vi "Waveform and Laser Controls V6.vi"() -> ()   [LabVIEW 2014]
uses:
  Waveform Scan Parameters.ctl
  <vilib>/Platform/TimedLoop/XDataNode/timing_clust.ctl
  <vilib>/Platform/TimedLoop/XDataNode/nitl_modes.ctl
  <vilib>/Platform/TimedLoop/XDataNode/wakeup.ctl
  <vilib>/rvi/Emulation/niFpgaGetClockAttributes.vi
  <vilib>/rvi/Emulation/niFpgaSctlEmulationGetInTimedLoop.vi
  <vilib>/rvi/Emulation/niFpgaEmulationReportErrorSimple.vi
  <vilib>/rvi/Emulation/niFpgaProcessEmulError.vi
  <vilib>/rvi/eio/common/nirviEmuTemplateMethod_errors.vi
  <vilib>/rvi/Emulation/niFpgaCriticalErrorInLSC.vi
  <vilib>/rvi/Memory/Memory_Emulation/nirvimemoryFastEmulation.vi
  <vilib>/rvi/Memory/Memory_Emulation/nirvimemoryEmulation.vi
  <vilib>/rvi/Emulation/niFpgaEmulationIsFPGAContextNoSignature.vi
  <vilib>/rvi/DataTransferAndStorage/Container/Common/niFpgaContainerGetUniqueNameForEmu.vi
  <vilib>/rvi/errors/nirviReportUnexpectedCaseInternalError (U32).vi
  <vilib>/rvi/Memory/Memory_Emulation/niFpgaMemoryEmulationCacheClearOnFirstRun.vi
  <vilib>/rvi/Memory/Memory_Emulation/nirvimemoryEmulationManagerCache_MakeExclusive.vi
  <vilib>/rvi/Memory/Memory_Emulation/niFpgaMemoryEmulationValidateCache.vi
  <vilib>/rvi/Memory/Memory_Emulation/nirvimemoryEmulationManagerCache_InsertValue.vi
  <vilib>/Utility/error.llb/Clear Errors.vi
  <vilib>/rvi/Memory/Memory_Emulation/nirvimemoryEmulationManagerCache_ReleaseExclusive.vi
  <vilib>/rvi/Memory/Memory_Emulation/nirvimemoryEmulationManagerCache_GetValue.vi
  <vilib>/rvi/Memory/Memory_Emulation/nirvimemoryEmulationManagerCache_SetValue.vi
  <vilib>/eio/EIONode/EIONode.xnode
  <vilib>/rvi/DataTransferAndStorage/Container/XNode/niFpgaContainer.xnode
  <vilib>/Platform/TimedLoop/XDataNode/XDataNode.xnode
  <vilib>/rvi/DataTransferAndStorage/Register/Emulation/niFpgaRegisterEmulation.vi
  <vilib>/Platform/TimedLoop/XDataNode/XDNodeRunTimeDep.lvlib
panel:
  in  "Current Frame":u8
  in  "Lower Shutter Command":bool
  in  "Upper Shutter Command":bool
  out "Lower Shutter Status":bool
  out "Upper Shutter Status":bool
  in  "stop":bool
  in  "775 AOM (I16)":i16=16500
  out "Laser Blank Trigger":bool
  in  "Laser On Time (Ticks)":u8=8
  in  "Sequences":u8=4
  in  "Laser Delay (Ticks)":u8
  in  "Laser States":u32
  in  "Blanking Off/Manual":bool
  in  "Z Piezo Axis":i16
  in  "Y Piezo Axis":i16
  in  "X Piezo Axis":i16
  out "End Linear Ramp":bool
  in  "End of Linear Ramp":u32
  in  "Z Stack Start Position (I16)":i16
  in  "Frames Per Z Step":u8
  in  "Number of Z Steps":u8
  in  "Z Step Size (I16)":i16
  in  "Stop Sync Signal":bool
  in  "Accums Per Line":u32[](array[numeric])=[0, 0, 0, 0]
  in  "Number of Lines":u32
  out "Frame Trigger":bool
  in  "Reset Position Error":bool
  in  "Galvo 1 Position (I16)":i16
  in  "Galvo 2 Position (I16)":i16
  in  "WF 3 Data Loaded":bool
  in  "WF 2 Data Loaded":bool
  in  "Waveform Scan Parameters":T1={"Scanning Mode"=0, "Fast Axis WF Length (Elements)"=0, "Fast Axis Sample Period (Ticks)"=40, "Slow Axis 1 WF Length (Elements)"=0, "Slow Axis 1 Sample Period (Ticks)"=40, "Slow Axis 1 Delay (25 ns) Steps"=40, "Slow Axis 2 WFLength (Elements)"=0, "Slow Axis 2 Sample Period (Ticks)"=40, "Slow Axis 2 Delay (25 ns) Steps"=40}
  in  "Resonant Mirror":T2
  in  "Galvo Mirror 2":T3
  in  "Galvo Mirror 1":T3
  in  "Start Waveforms":bool
  in  "Unused Axis Offset":i16
  in  "Slow Axis 2 Waveform Element":i16
  in  "Fast Axis Waveform Element":i16
  in  "Slow Axis 1 Waveform Element":i16
  in  "WF 1 Data Loaded":bool
  # "V2 - Adding in a line clock\nV3 - Cluster Scan Parameters"
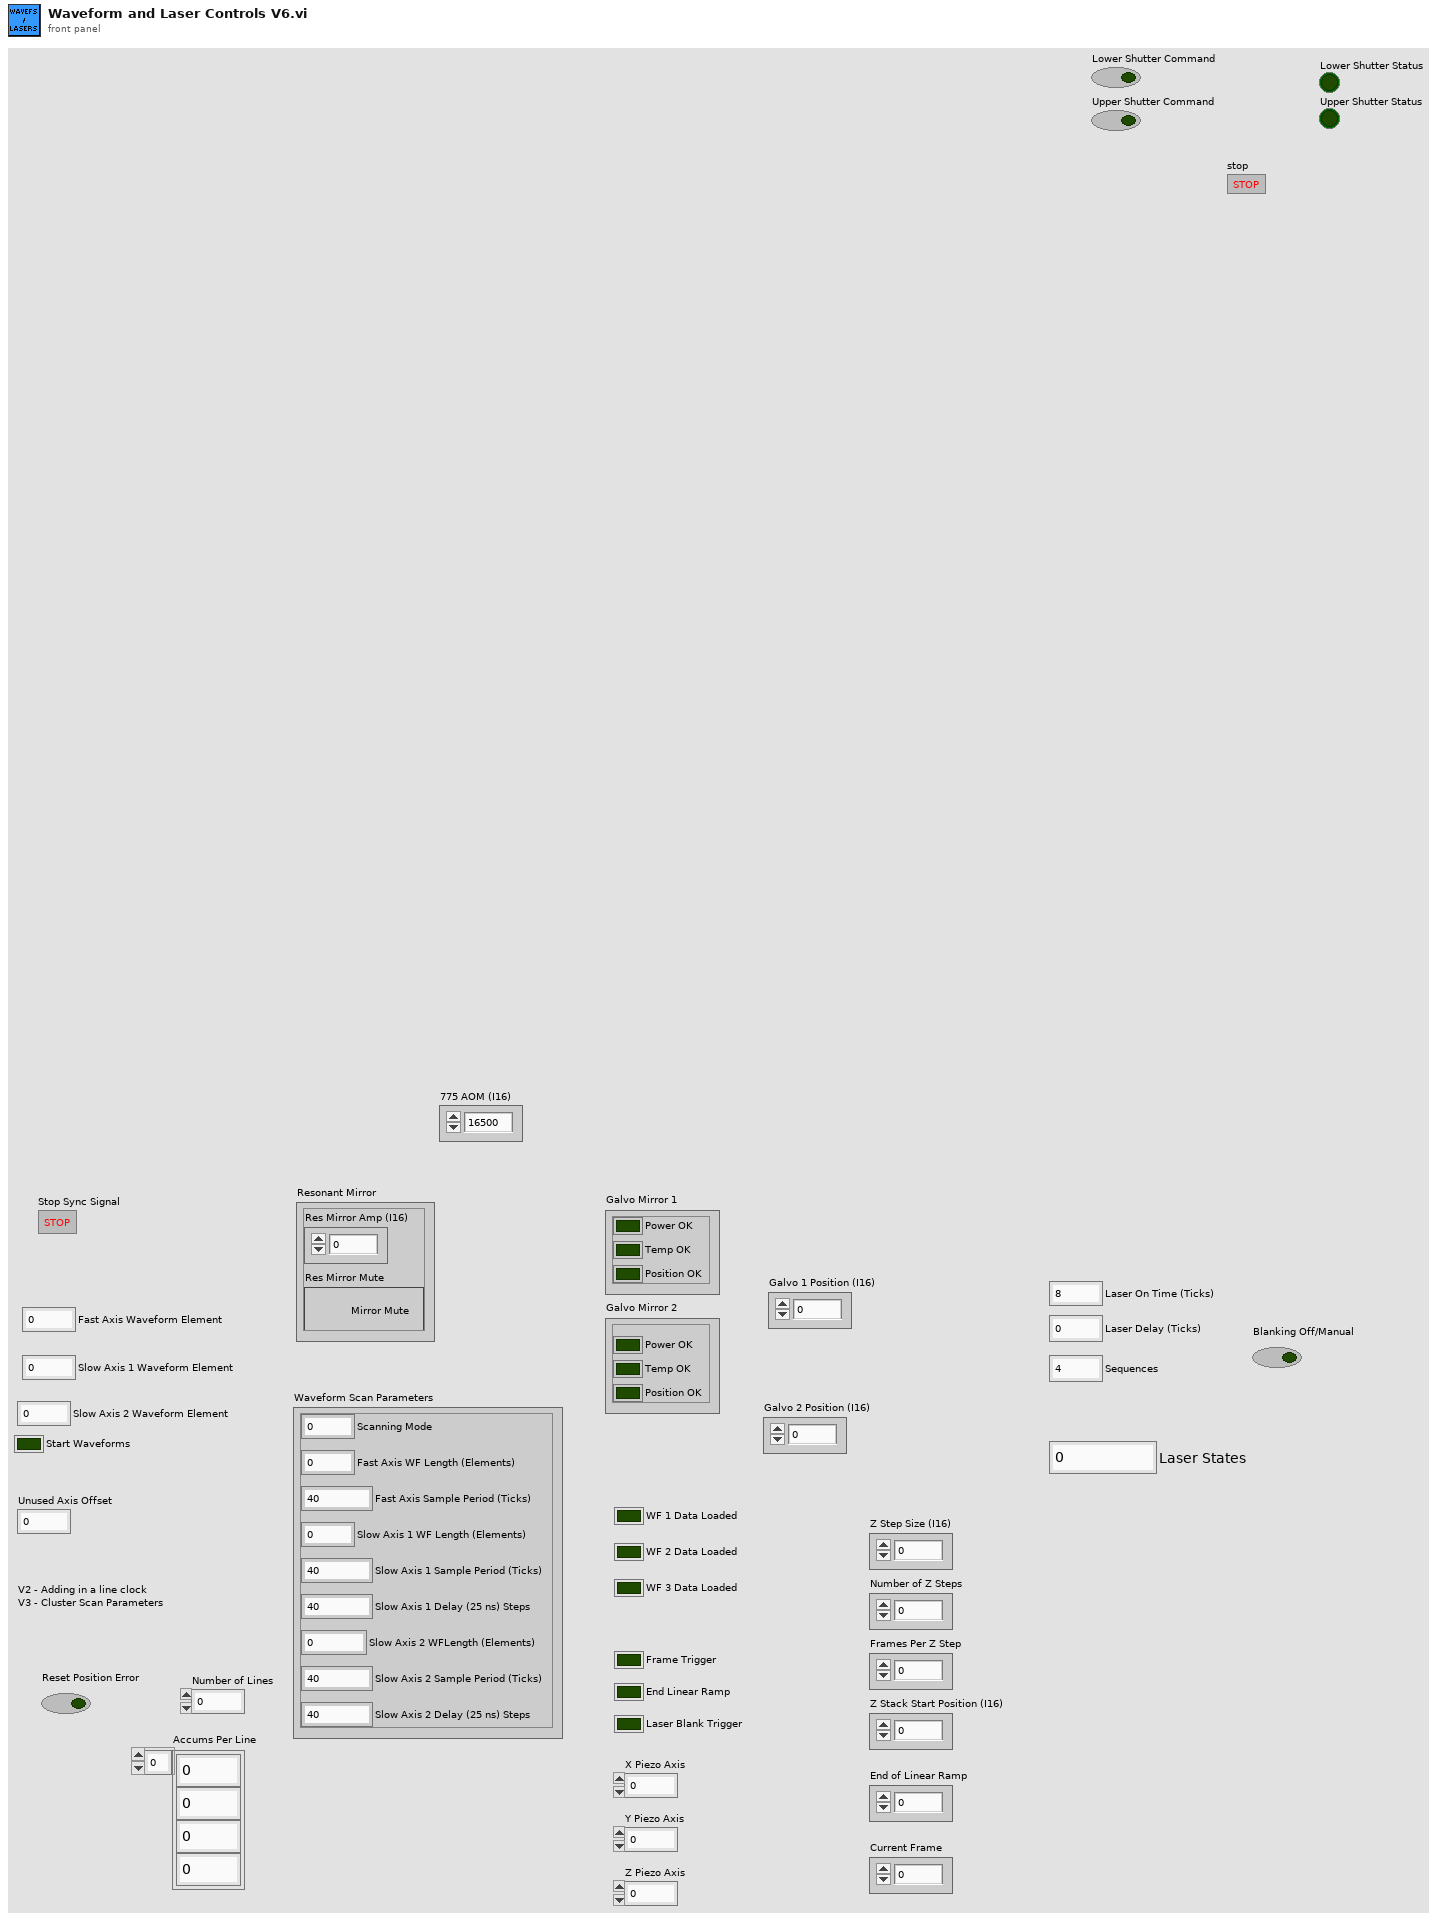
[diagram p1: front panel]
types:
  T1 = typedef "Waveform Scan Parameters.ctl" = cluster{"Scanning Mode":u8, "Fast Axis WF Length (Elements)":i32, "Fast Axis Sample Period (Ticks)":u32, "Slow Axis 1 WF Length (Elements)":i32, "Slow Axis 1 Sample Period (Ticks)":u32, "Slow Axis 1 Delay (25 ns) Steps":i32, "Slow Axis 2 WFLength (Elements)":i32, "Slow Axis 2 Sample Period (Ticks)":u32, "Slow Axis 2 Delay (25 ns) Steps":i32}
  T2 = cluster{"Res Mirror Amp (I16)":i16, "Res Mirror Mute":bool}
  T3 = cluster{"Power OK":bool, "Temp OK":bool, "Position OK":bool}
  T4 = typedef "XDNodeRunTimeDep.lvlib/timing_clust.ctl" = cluster{"Expected End [f-1]":u64, "Actual End [f-1]":u64, "Finished Late? [f-1]":bool, "Expected End [i-1]":u64, "Actual End [i-1]":u64, "Finished Late? [i-1]":bool, "Expected Start [i]":u64, "Actual Start [i]":u64, "Expected Start [f]":u64, "Actual Start [f]":u64, "Source Name":string, "Structure Name":string, "Period":i64, "Deadline":i64, "Offset":i64, "Start":i64, "Priority":i32, "Timeout":i32, "Mode":T5, "Wakeup Reason":T6, "Error":errorcluster, "Source Type":string, "Secondary Source Type":string, "Global End Time":u64, "Global Start Time":u64, "Frame Duration":u64, "Iteration Duration":u64, "Assigned CPU":i32, "I/O Scan Engine Mode":u32}
  T5 = typedef "XDNodeRunTimeDep.lvlib/nitl_modes.ctl" = enum32{"No Change", "Process missed periods, maintain original phase", "Discard missed periods, maintain original phase", "Process missed periods, ignore original phase", "Discard missed periods, ignore original phase"}
  T6 = typedef "XDNodeRunTimeDep.lvlib/wakeup.ctl" = enum32{"Normal", "Aborted", "Asynchronous wakeup", "Timing source error", "Timed loop error", "Timeout"}
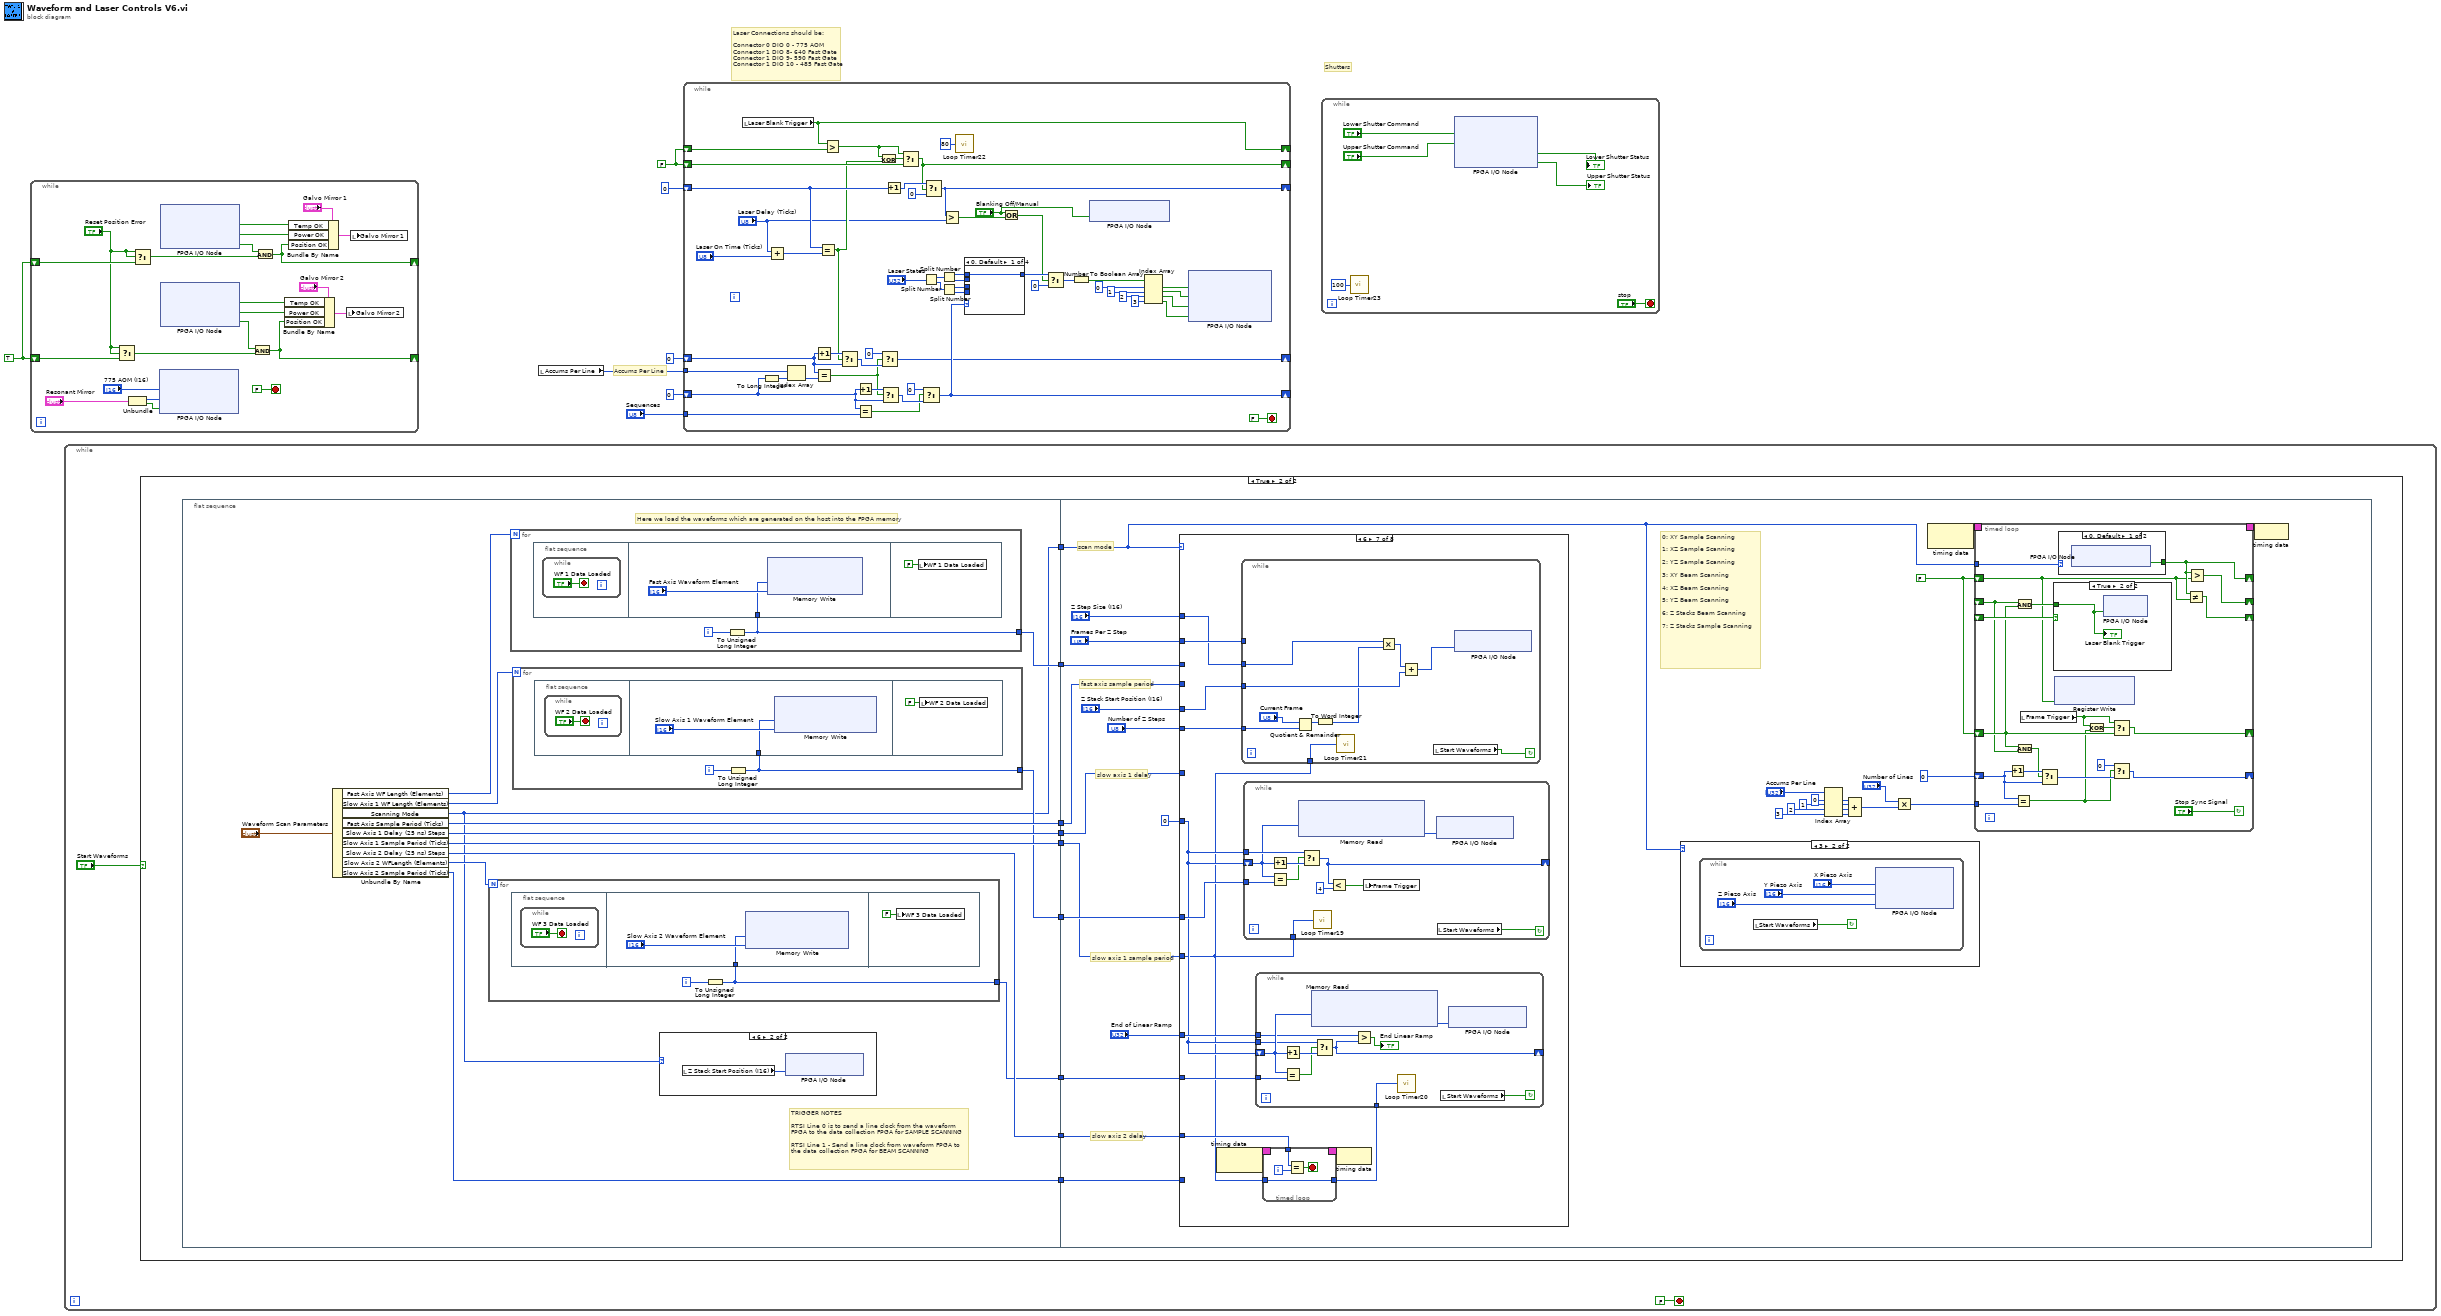
[diagram p0: block diagram]
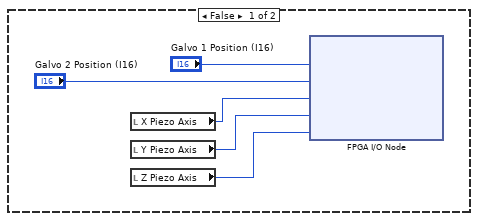
[diagram p5: hidden frame]
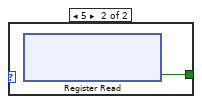
[diagram p7: hidden frame]
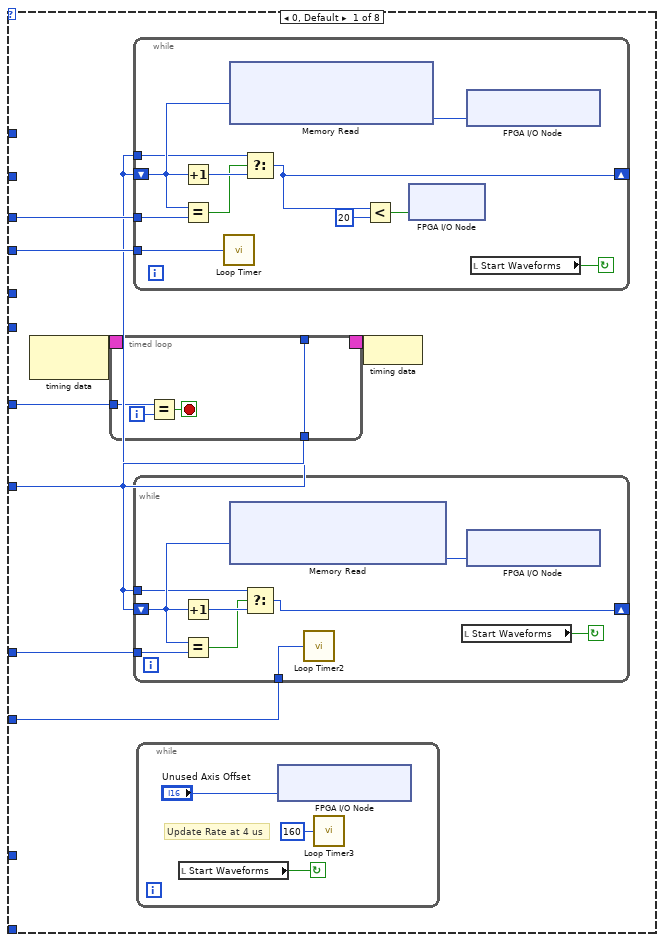
[diagram p10: hidden frame]
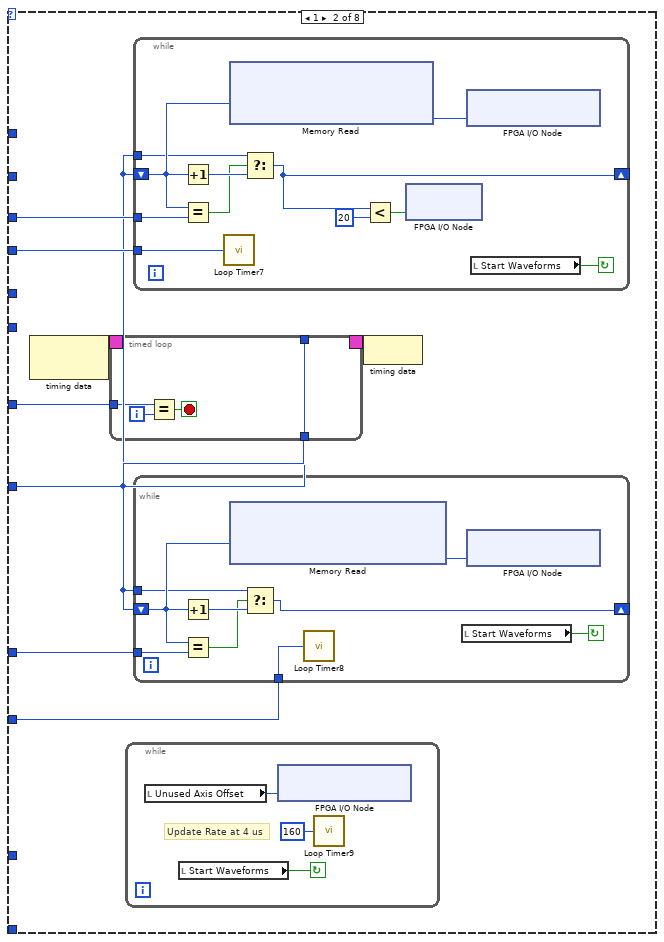
[diagram p11: hidden frame]
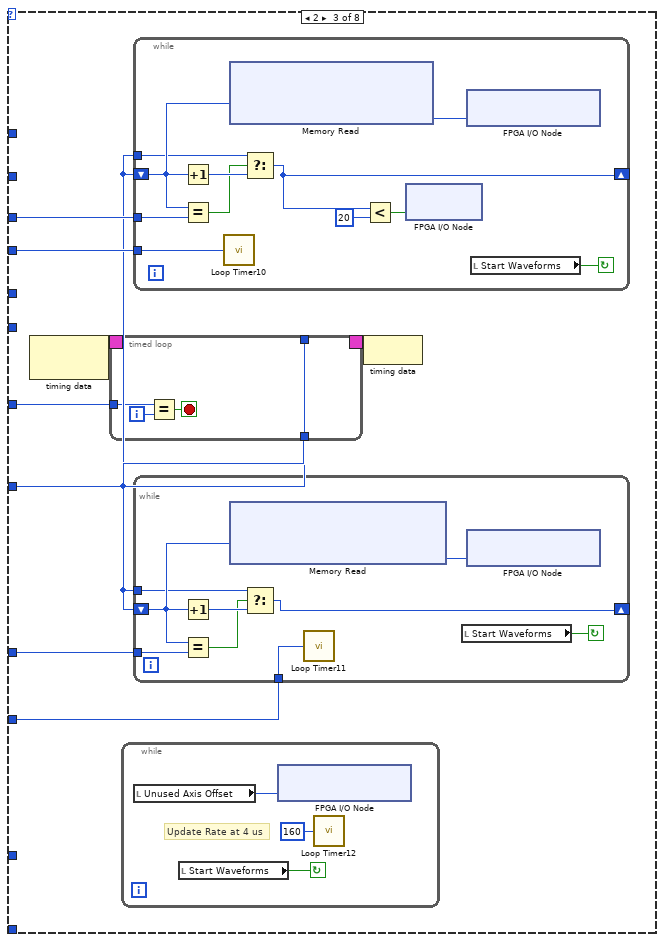
[diagram p12: hidden frame]
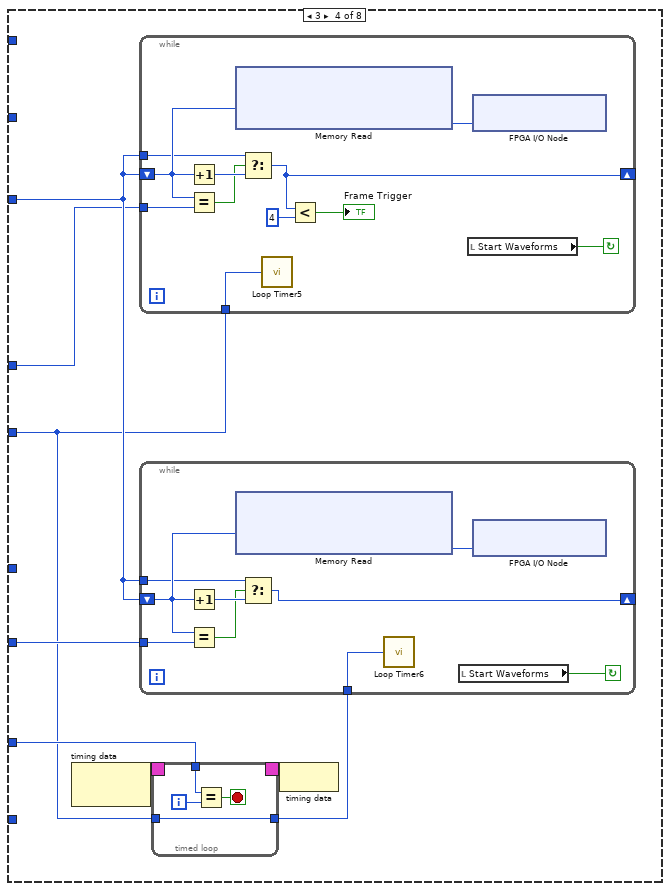
[diagram p13: hidden frame]
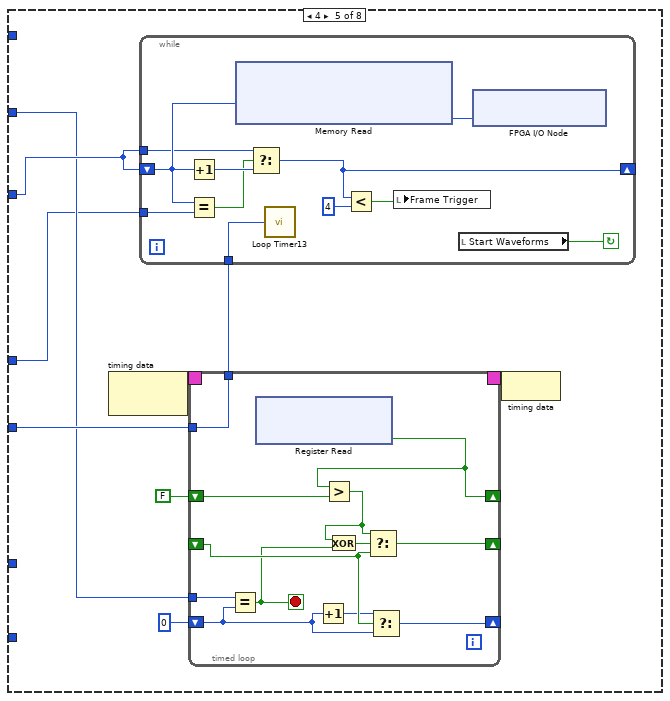
[diagram p14: hidden frame]
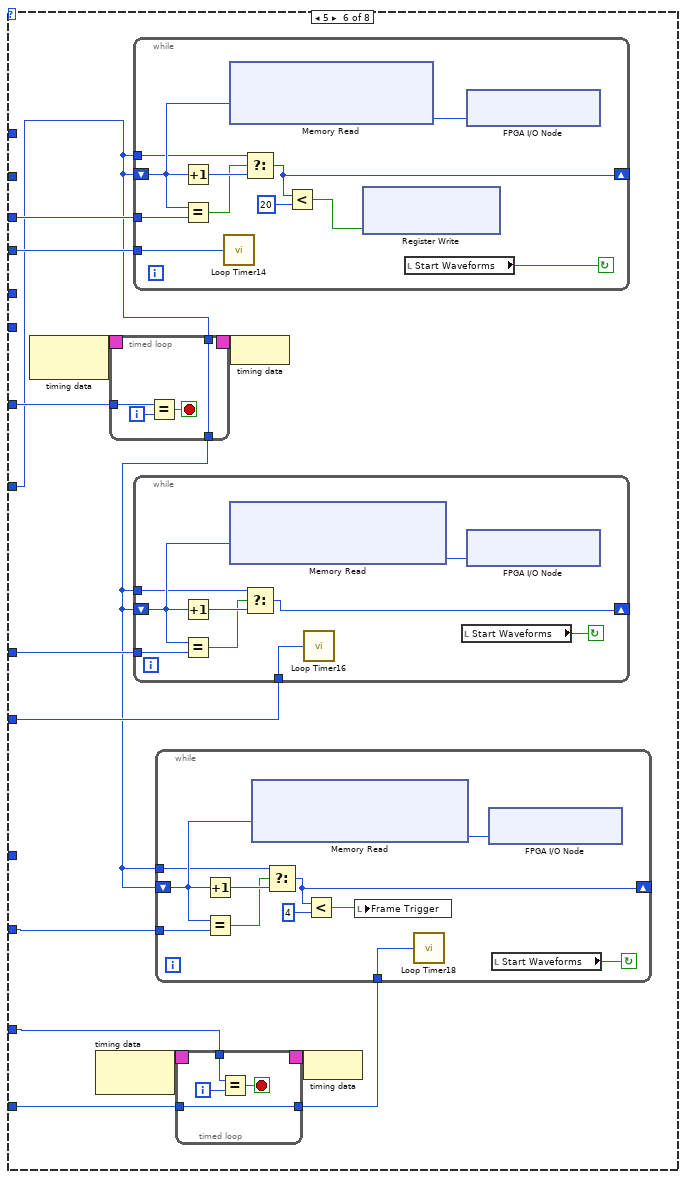
[diagram p15: hidden frame]
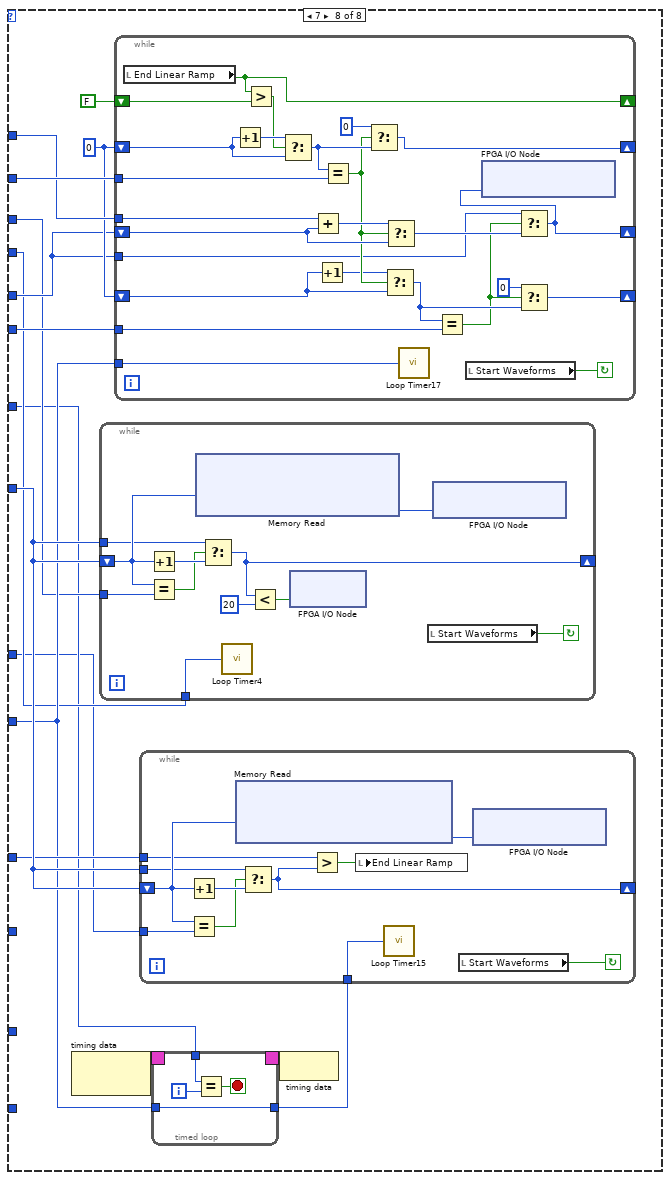
[diagram p16: hidden frame]
diagram:
  w2 = FALSE
  w7 = TRUE
  # "Shutters"
  # "Laser Connections should be:\n\nConnector 0 DIO 0 - 775 AOM\nConnector 1 DIO 8- 640 Fast Gate\nConnector 1 DIO 9- 590 Fast Gate\nConnector 1 DIO 10 - 485 Fast Gate"
  # "Accums Per Line"
  n1 = while {
    shift-right: [w15] -> _
    shift-left: w7 -> [w17]
    shift-right: [w11] -> _
    shift-left: w7 -> [w13]
    stop <- FALSE stop-if-true
    n2 = Select(t="Reset Position Error", s="Reset Position Error", f=w17) -> (s? t:f=w16:bool)
    n3 = Unbundle("Resonant Mirror") -> ("Res Mirror Amp (I16)"=w27:i16, "Res Mirror Mute"=w26:bool)
    n4 = Select(t="Reset Position Error", s="Reset Position Error", f=w13) -> (s? t:f=w12:bool)
    n5 = xnode "FPGA I/O Node"("Connector0/AO4"="775 AOM (I16)", "Connector0/AO7"=w27, "Connector0/DIO7"=w26) -> ()  [unwired: 4 in, 4 out]
    n6 = xnode "FPGA I/O Node"() -> ("Connector0/DIO1"=w8:bool, "Connector0/DIO2"=w25:bool, "Connector0/DIO3"=w14:bool)  [unwired: 4 in, 4 out]
    n7 = xnode "FPGA I/O Node"() -> ("Connector0/DIO4"=w19:bool, "Connector0/DIO5"=w20:bool, "Connector0/DIO6"=w18:bool)  [unwired: 4 in, 4 out]
    n8 = And(x=w18, y=w16) -> (x .and. y?=w15:bool)
    n9 = And(x=w14, y=w12) -> (x .and. y?=w11:bool)
    n10 = Bundle By Name(cluster="Galvo Mirror 2", "Temp OK"=w19, "Power OK"=w20, "Position OK"=w15) -> (w22:T3)
    n11 = Bundle By Name(cluster="Galvo Mirror 1", "Temp OK"=w8, "Power OK"=w25, "Position OK"=w11) -> (w24:T3)
    n12 = local write "Galvo Mirror 2"(w22) -> ()
    n13 = local write "Galvo Mirror 1"(w24) -> ()
  }
  n14 = while {
    stop <- FALSE stop-if-true
    n15 = case shown="True" "Start Waveforms" {
      frame False {
        n16 = local read "X Piezo Axis"() -> (w34:i16)
        n17 = local read "Y Piezo Axis"() -> (w33:i16)
        n18 = local read "Z Piezo Axis"() -> (w32:i16)
        n19 = xnode "FPGA I/O Node"("Connector0/AO5"="Galvo 1 Position (I16)", "Connector0/AO6"="Galvo 2 Position (I16)", "Connector0/AO1"=w34, "Connector0/AO2"=w33, "Connector0/AO3"=w32) -> ()  [unwired: 5 in, 5 out]
      }
      frame True {
        n20 = flat-sequence {
          tunnel: [w58] -> w45
          tunnel: [w48] -> w44
          tunnel: [w49] -> w43
          tunnel: [w47] -> w42
          tunnel: [w56] -> w41
          tunnel: [w55] -> w40
          tunnel: [w54] -> w39
          tunnel: [w53] -> w38
          tunnel: [w46] -> w37
          tunnel: w45 -> [w108]
          tunnel: w44 -> [w107]
          tunnel: w43 -> [w105]
          tunnel: w42 -> [w79]
          tunnel: w41 -> [w104]
          tunnel: w40 -> [w103]
          tunnel: w39 -> [w102]
          tunnel: w38 -> [w101]
          tunnel: w37 -> [w78]
          frame #0 {
            # "TRIGGER NOTES\n\nRTSI Line 0 is to send a line clock from the waveform\nFPGA to the data collection FPGA for SAMPLE SCANNING\n\nRTSI Line 1 - Send a line clock from waveform FPGA to\nthe data collection FPGA for BEAM SCANNING"
            # "Here we load the waveforms which are generated on the host into the FPGA memory"
            n21 = Unbundle By Name("Waveform Scan Parameters") -> ("Fast Axis WF Length (Elements)"=w52:i32, "Slow Axis 1 WF Length (Elements)"=w51:i32, "Scanning Mode"=w47:u8, "Fast Axis Sample Period (Ticks)"=w56:u32, "Slow Axis 1 Delay (25 ns) Steps"=w55:i32, "Slow Axis 1 Sample Period (Ticks)"=w54:u32, "Slow Axis 2 Delay (25 ns) Steps"=w53:i32, "Slow Axis 2 WFLength (Elements)"=w50:i32, "Slow Axis 2 Sample Period (Ticks)"=w46:u32)
            n22 = for {
              N: w50 -> [_]
              tunnel: [w60] -> w48
              i -> [w61]
              n23 = flat-sequence {
                tunnel: w60 -> [w63]
                frame #0 {
                  n24 = while {
                    stop <- "WF 3 Data Loaded" stop-if-true
                  }
                }
                frame #1 {
                  n25 = xnode ("Memory Write")("Address"=w63, "Data"="Slow Axis 2 Waveform Element") -> ()  [unwired: 1 in, 1 out]
                }
                frame #2 {
                  n26 = local write "WF 3 Data Loaded"(FALSE ("Host Data Loaded")) -> ()
                }
              }
              n27 = To Unsigned Long Integer(number=w61) -> (unsigned 32bit integer=w60:u32)
            }
            n28 = for {
              N: w52 -> [_]
              tunnel: [w72] -> w58
              i -> [w73]
              n29 = flat-sequence {
                tunnel: w72 -> [w75]
                frame #0 {
                  n30 = while {
                    stop <- "WF 1 Data Loaded" stop-if-true
                  }
                }
                frame #1 {
                  n31 = xnode ("Memory Write")("Address"=w75, "Data"="Fast Axis Waveform Element") -> ()  [unwired: 1 in, 1 out]
                }
                frame #2 {
                  n32 = local write "WF 1 Data Loaded"(FALSE ("Host Data Loaded")) -> ()
                }
              }
              n33 = To Unsigned Long Integer(number=w73) -> (unsigned 32bit integer=w72:u32)
            }
            n34 = for {
              N: w51 -> [_]
              tunnel: [w66] -> w49
              i -> [w67]
              n35 = flat-sequence {
                tunnel: w66 -> [w69]
                frame #0 {
                  n36 = while {
                    stop <- "WF 2 Data Loaded" stop-if-true
                  }
                }
                frame #1 {
                  n37 = xnode ("Memory Write")("Address"=w69, "Data"="Slow Axis 1 Waveform Element") -> ()  [unwired: 1 in, 1 out]
                }
                frame #2 {
                  n38 = local write "WF 2 Data Loaded"(FALSE ("Host Data Loaded")) -> ()
                }
              }
              n39 = To Unsigned Long Integer(number=w67) -> (unsigned 32bit integer=w66:u32)
            }
            n40 = case shown="6" w47 {
              frame 0, Default {
              }
              frame 6 {
                n41 = local read "Z Stack Start Position (I16)"() -> (w59:i16)
                n42 = xnode "FPGA I/O Node"("Connector0/AO3"=w59) -> ()  [unwired: 1 in, 1 out]
              }
            }
          }
          frame #1 {
            w81 = FALSE
            # "slow axis 2 delay"
            # "slow axis 1 sample period"
            # "slow axis 1 delay"
            # "fast axis sample period"
            # "scan mode"
            # "0: XY Sample Scanning\n\n1: XZ Sample Scanning\n\n2: YZ Sample Scanning\n\n3: XY Beam Scanning\n\n4: XZ Beam Scanning\n\n5: YZ Beam Scanning\n\n6: Z Stacks Beam Scanning\n\n7: Z Stacks Sample Scanning"
            n43 = case shown="6" w79 {
              tunnel: w108 -> [w147 w187 w227 _ _ w347 _ w450]
              tunnel: w104 -> [w146 w186 w226 _ _ w346 _ w451]
              tunnel: w107 -> [_ _ _ w268 _ w341 w407 _]
              tunnel: u32 0 -> [w141 w181 w221 w267 w305 w343 w397 w463]
              tunnel: w103 -> [w145 w185 w225 _ w303 w345 _ w449]
              tunnel: w101 -> [_ _ _ w266 _ w340 w406 _]
              tunnel: w105 -> [w143 w183 w223 w261 w302 w344 w403 w448]
              tunnel: w102 -> [w142 w182 w222 w262 w304 w342 w395 w452]
              tunnel: "Frames Per Z Step" -> [_ _ _ _ _ _ w402 w459]
              tunnel: "Z Stack Start Position (I16)" -> [_ _ _ _ _ _ w398 w455]
              tunnel: "Z Step Size (I16)" -> [_ _ _ _ _ _ w401 w458]
              tunnel: "Number of Z Steps" -> [_ _ _ _ _ _ w400 w456]
              tunnel: "End of Linear Ramp" -> [_ _ _ _ _ _ w399 w454]
              tunnel: w78 -> [_ _ _ _ _ w333 _ _]
              frame 0, Default {
                n44 = node-c288() -> (w149:T4)  [unwired: 1 in]
                n45 = timed-loop {
                  timing: w149 -> [_]
                  timing-out: [_] -> w148
                  tunnel: w145 -> [w154]
                  tunnel: w141 -> [w153]
                  tunnel: [w153] -> w144
                  i -> [w156]
                  stop <- w155 stop-if-true
                  n46 = Equal?(x=w154, y=w156) -> (x = y?=w155:bool)
                }
                n47 = while {
                  shift-right: [w172] -> _
                  shift-left: w141 -> [w178]
                  tunnel: w147 -> [w179]
                  tunnel: w146 -> [w176]
                  tunnel: w141 -> [w175]
                  stop <- w174 continue-if-true
                  n48 = Increment(x=w178) -> (x+1=w180:u32)
                  n49 = Equal?(x=w178, y=w179) -> (x = y?=w173:bool)
                  n50 = call "Loop Timer"("Count(Ticks)"=w176) -> ()  [unwired: 1 out]
                  n51 = xnode ("Memory Read")("Address"=w178) -> ("Data"=w177:i16)  [unwired: 1 in, 1 out]
                  n52 = Select(t=w175, s=w173, f=w180) -> (s? t:f=w172:u32)
                  n53 = Less?(x=w172, y=u32 20) -> (x < y?=w170:bool)
                  n54 = xnode "FPGA I/O Node"("TRIG0"=w170) -> ()  [unwired: 1 in, 1 out]
                  n55 = xnode "FPGA I/O Node"("Connector0/AO1"=w177) -> ()  [unwired: 1 in, 1 out]
                  n56 = local read "Start Waveforms"() -> (w174:bool)
                }
                n57 = while {
                  shift-right: [w168] -> _
                  shift-left: w144 -> [w165]
                  tunnel: w143 -> [w167]
                  tunnel: w144 -> [w163]
                  tunnel: w142 -> [w162]
                  stop <- w161 continue-if-true
                  n58 = Increment(x=w165) -> (x+1=w169:u32)
                  n59 = Equal?(x=w165, y=w167) -> (x = y?=w166:bool)
                  n60 = xnode ("Memory Read")("Address"=w165) -> ("Data"=w164:i16)  [unwired: 1 in, 1 out]
                  n61 = Select(t=w163, s=w166, f=w169) -> (s? t:f=w168:u32)
                  n62 = call "Loop Timer2"("Count(Ticks)"=w162) -> ()  [unwired: 1 out]
                  n63 = local read "Start Waveforms"() -> (w161:bool)
                  n64 = xnode "FPGA I/O Node"("Connector0/AO2"=w164) -> ()  [unwired: 1 in, 1 out]
                }
                n65 = while {
                  stop <- w150 continue-if-true
                  # "Update Rate at 4 us"
                  n66 = local read "Start Waveforms"() -> (w150:bool)
                  n67 = xnode "FPGA I/O Node"("Connector0/AO3"="Unused Axis Offset") -> ()  [unwired: 1 in, 1 out]
                  n68 = call "Loop Timer3"("Count(Ticks)"=u32 160) -> ()  [unwired: 1 out]
                }
                n69 = node-c288(w148) -> ()
              }
              frame 1 {
                n70 = node-c288() -> (w189:T4)  [unwired: 1 in]
                n71 = timed-loop {
                  timing: w189 -> [_]
                  timing-out: [_] -> w188
                  tunnel: w185 -> [w194]
                  tunnel: w181 -> [w193]
                  tunnel: [w193] -> w184
                  i -> [w196]
                  stop <- w195 stop-if-true
                  n72 = Equal?(x=w194, y=w196) -> (x = y?=w195:bool)
                }
                n73 = while {
                  stop <- w191 continue-if-true
                  # "Update Rate at 4 us"
                  n74 = local read "Unused Axis Offset"() -> (w190:i16)
                  n75 = local read "Start Waveforms"() -> (w191:bool)
                  n76 = xnode "FPGA I/O Node"("Connector0/AO2"=w190) -> ()  [unwired: 1 in, 1 out]
                  n77 = call "Loop Timer9"("Count(Ticks)"=u32 160) -> ()  [unwired: 1 out]
                }
                n78 = while {
                  shift-right: [w212] -> _
                  shift-left: w181 -> [w218]
                  tunnel: w187 -> [w219]
                  tunnel: w186 -> [w216]
                  tunnel: w181 -> [w215]
                  stop <- w214 continue-if-true
                  n79 = Increment(x=w218) -> (x+1=w220:u32)
                  n80 = Equal?(x=w218, y=w219) -> (x = y?=w213:bool)
                  n81 = call "Loop Timer7"("Count(Ticks)"=w216) -> ()  [unwired: 1 out]
                  n82 = xnode ("Memory Read")("Address"=w218) -> ("Data"=w217:i16)  [unwired: 1 in, 1 out]
                  n83 = Select(t=w215, s=w213, f=w220) -> (s? t:f=w212:u32)
                  n84 = Less?(x=w212, y=u32 20) -> (x < y?=w210:bool)
                  n85 = xnode "FPGA I/O Node"("TRIG0"=w210) -> ()  [unwired: 1 in, 1 out]
                  n86 = xnode "FPGA I/O Node"("Connector0/AO1"=w217) -> ()  [unwired: 1 in, 1 out]
                  n87 = local read "Start Waveforms"() -> (w214:bool)
                }
                n88 = while {
                  shift-right: [w208] -> _
                  shift-left: w184 -> [w205]
                  tunnel: w183 -> [w207]
                  tunnel: w184 -> [w203]
                  tunnel: w182 -> [w202]
                  stop <- w201 continue-if-true
                  n89 = Increment(x=w205) -> (x+1=w209:u32)
                  n90 = Equal?(x=w205, y=w207) -> (x = y?=w206:bool)
                  n91 = xnode ("Memory Read")("Address"=w205) -> ("Data"=w204:i16)  [unwired: 1 in, 1 out]
                  n92 = Select(t=w203, s=w206, f=w209) -> (s? t:f=w208:u32)
                  n93 = call "Loop Timer8"("Count(Ticks)"=w202) -> ()  [unwired: 1 out]
                  n94 = local read "Start Waveforms"() -> (w201:bool)
                  n95 = xnode "FPGA I/O Node"("Connector0/AO3"=w204) -> ()  [unwired: 1 in, 1 out]
                }
                n96 = node-c288(w188) -> ()
              }
              frame 2 {
                n97 = node-c288() -> (w229:T4)  [unwired: 1 in]
                n98 = timed-loop {
                  timing: w229 -> [_]
                  timing-out: [_] -> w228
                  tunnel: w225 -> [w234]
                  tunnel: w221 -> [w233]
                  tunnel: [w233] -> w224
                  i -> [w236]
                  stop <- w235 stop-if-true
                  n99 = Equal?(x=w234, y=w236) -> (x = y?=w235:bool)
                }
                n100 = while {
                  stop <- w231 continue-if-true
                  # "Update Rate at 4 us"
                  n101 = local read "Unused Axis Offset"() -> (w230:i16)
                  n102 = local read "Start Waveforms"() -> (w231:bool)
                  n103 = xnode "FPGA I/O Node"("Connector0/AO1"=w230) -> ()  [unwired: 1 in, 1 out]
                  n104 = call "Loop Timer12"("Count(Ticks)"=u32 160) -> ()  [unwired: 1 out]
                }
                n105 = while {
                  shift-right: [w252] -> _
                  shift-left: w221 -> [w258]
                  tunnel: w227 -> [w259]
                  tunnel: w226 -> [w256]
                  tunnel: w221 -> [w255]
                  stop <- w254 continue-if-true
                  n106 = Increment(x=w258) -> (x+1=w260:u32)
                  n107 = Equal?(x=w258, y=w259) -> (x = y?=w253:bool)
                  n108 = call "Loop Timer10"("Count(Ticks)"=w256) -> ()  [unwired: 1 out]
                  n109 = xnode ("Memory Read")("Address"=w258) -> ("Data"=w257:i16)  [unwired: 1 in, 1 out]
                  n110 = Select(t=w255, s=w253, f=w260) -> (s? t:f=w252:u32)
                  n111 = Less?(x=w252, y=u32 20) -> (x < y?=w250:bool)
                  n112 = xnode "FPGA I/O Node"("TRIG0"=w250) -> ()  [unwired: 1 in, 1 out]
                  n113 = xnode "FPGA I/O Node"("Connector0/AO2"=w257) -> ()  [unwired: 1 in, 1 out]
                  n114 = local read "Start Waveforms"() -> (w254:bool)
                }
                n115 = while {
                  shift-right: [w248] -> _
                  shift-left: w224 -> [w245]
                  tunnel: w223 -> [w247]
                  tunnel: w224 -> [w243]
                  tunnel: w222 -> [w242]
                  stop <- w241 continue-if-true
                  n116 = Increment(x=w245) -> (x+1=w249:u32)
                  n117 = Equal?(x=w245, y=w247) -> (x = y?=w246:bool)
                  n118 = xnode ("Memory Read")("Address"=w245) -> ("Data"=w244:i16)  [unwired: 1 in, 1 out]
                  n119 = Select(t=w243, s=w246, f=w249) -> (s? t:f=w248:u32)
                  n120 = call "Loop Timer11"("Count(Ticks)"=w242) -> ()  [unwired: 1 out]
                  n121 = local read "Start Waveforms"() -> (w241:bool)
                  n122 = xnode "FPGA I/O Node"("Connector0/AO3"=w244) -> ()  [unwired: 1 in, 1 out]
                }
                n123 = node-c288(w228) -> ()
              }
              frame 3 {
                n124 = node-c288() -> (w265:T4)  [unwired: 1 in]
                n125 = while {
                  shift-right: [w288] -> _
                  shift-left: w267 -> [w294]
                  tunnel: w261 -> [w295]
                  tunnel: w262 -> [w292]
                  tunnel: w267 -> [w291]
                  stop <- w290 continue-if-true
                  n126 = Increment(x=w294) -> (x+1=w296:u32)
                  n127 = Equal?(x=w294, y=w295) -> (x = y?=w289:bool)
                  n128 = xnode ("Memory Read")("Address"=w294) -> ("Data"=w293:i16)  [unwired: 1 in, 1 out]
                  n129 = Select(t=w291, s=w289, f=w296) -> (s? t:f=w288:u32)
                  n130 = call "Loop Timer5"("Count(Ticks)"=w292) -> ()  [unwired: 1 out]
                  n131 = Less?(x=w288, y=u32 4) -> (x < y?=→"Frame Trigger":bool)
                  n132 = local read "Start Waveforms"() -> (w290:bool)
                  n133 = xnode "FPGA I/O Node"("Connector0/AO5"=w293) -> ()  [unwired: 1 in, 1 out]
                }
                n134 = timed-loop {
                  timing: w265 -> [_]
                  timing-out: [_] -> w264
                  tunnel: w262 -> [w278]
                  tunnel: [w278] -> w263
                  tunnel: w266 -> [w279]
                  i -> [w281]
                  stop <- w280 stop-if-true
                  n135 = Equal?(x=w279, y=w281) -> (x = y?=w280:bool)
                }
                n136 = while {
                  shift-right: [w276] -> _
                  shift-left: w267 -> [w274]
                  tunnel: w268 -> [w275]
                  tunnel: w263 -> [w272]
                  tunnel: w267 -> [w271]
                  stop <- w270 continue-if-true
                  n137 = Increment(x=w274) -> (x+1=w277:u32)
                  n138 = Equal?(x=w274, y=w275) -> (x = y?=w269:bool)
                  n139 = xnode ("Memory Read")("Address"=w274) -> ("Data"=w273:i16)  [unwired: 1 in, 1 out]
                  n140 = Select(t=w271, s=w269, f=w277) -> (s? t:f=w276:u32)
                  n141 = call "Loop Timer6"("Count(Ticks)"=w272) -> ()  [unwired: 1 out]
                  n142 = local read "Start Waveforms"() -> (w270:bool)
                  n143 = xnode "FPGA I/O Node"("Connector0/AO6"=w273) -> ()  [unwired: 1 in, 1 out]
                }
                n144 = node-c288(w264) -> ()
              }
              frame 4 {
                n145 = node-c288() -> (w300:T4)  [unwired: 1 in]
                n146 = timed-loop {
                  timing: w300 -> [_]
                  timing-out: [_] -> w299
                  tunnel: w304 -> [w308]
                  shift-right: [w306] -> _
                  shift-left: FALSE -> [w317]
                  shift-right: [w314] -> _
                  shift-left: _ -> [w313]
                  shift-right: [w311] -> _
                  shift-left: 0 -> [w309]
                  tunnel: w303 -> [w310]
                  tunnel: [w308] -> w301
                  stop <- w307 stop-if-true
                  n147 = Equal?(x=w310, y=w309) -> (x = y?=w307:bool)
                  n148 = xnode ("Register Read")() -> ("Data"=w306:bool)  [unwired: 1 in, 1 out]
                  n149 = Increment(x=w309) -> (x+1=w312:i32)
                  n150 = Greater?(x=w306, y=w317) -> (0:w315:bool)
                  n151 = Exclusive Or(1:w307, 2:w315) -> (0:w316:bool)
                  n152 = Select(t=w315, s=w316, f=w313) -> (s? t:f=w314:bool)
                  n153 = Select(t=w312, s=w313, f=w309) -> (s? t:f=w311:i32)
                }
                n154 = while {
                  shift-right: [w323] -> _
                  shift-left: w305 -> [w329]
                  tunnel: w302 -> [w331]
                  tunnel: w301 -> [w327]
                  tunnel: w305 -> [w326]
                  stop <- w325 continue-if-true
                  n155 = Increment(x=w329) -> (x+1=w332:u32)
                  n156 = Equal?(x=w329, y=w331) -> (x = y?=w330:bool)
                  n157 = xnode ("Memory Read")("Address"=w329) -> ("Data"=w328:i16)  [unwired: 1 in, 1 out]
                  n158 = Select(t=w326, s=w330, f=w332) -> (s? t:f=w323:u32)
                  n159 = call "Loop Timer13"("Count(Ticks)"=w327) -> ()  [unwired: 1 out]
                  n160 = Less?(x=w323, y=u32 4) -> (x < y?=w322:bool)
                  n161 = local write "Frame Trigger"(w322) -> ()
                  n162 = local read "Start Waveforms"() -> (w325:bool)
                  n163 = xnode "FPGA I/O Node"("Connector0/AO3"=w328) -> ()  [unwired: 1 in, 1 out]
                }
                n164 = node-c288(w299) -> ()
              }
              frame 5 {
                n165 = node-c288() -> (w339:T4)  [unwired: 1 in]
                n166 = node-c288() -> (w337:T4)  [unwired: 1 in]
                n167 = timed-loop {
                  timing: w339 -> [_]
                  timing-out: [_] -> w338
                  tunnel: w345 -> [w368]
                  tunnel: w343 -> [w367]
                  tunnel: [w367] -> w334
                  i -> [w370]
                  stop <- w369 stop-if-true
                  n168 = Equal?(x=w368, y=w370) -> (x = y?=w369:bool)
                }
                n169 = while {
                  shift-right: [w387] -> _
                  shift-left: w343 -> [w392]
                  tunnel: w347 -> [w393]
                  tunnel: w346 -> [w390]
                  tunnel: w343 -> [w389]
                  stop <- w385 continue-if-true
                  n170 = Increment(x=w392) -> (x+1=w394:u32)
                  n171 = Equal?(x=w392, y=w393) -> (x = y?=w388:bool)
                  n172 = call "Loop Timer14"("Count(Ticks)"=w390) -> ()  [unwired: 1 out]
                  n173 = xnode ("Memory Read")("Address"=w392) -> ("Data"=w391:i16)  [unwired: 1 in, 1 out]
                  n174 = Select(t=w389, s=w388, f=w394) -> (s? t:f=w387:u32)
                  n175 = Less?(x=w387, y=u32 20) -> (x < y?=w384:bool)
                  n176 = xnode ("Register Write")("Data"=w384) -> ()  [unwired: 1 in, 1 out]
                  n177 = local read "Start Waveforms"() -> (w385:bool)
                  n178 = xnode "FPGA I/O Node"("Connector0/AO5"=w391) -> ()  [unwired: 1 in, 1 out]
                }
                n179 = while {
                  shift-right: [w382] -> _
                  shift-left: w334 -> [w379]
                  tunnel: w344 -> [w381]
                  tunnel: w334 -> [w377]
                  tunnel: w342 -> [w376]
                  stop <- w375 continue-if-true
                  n180 = Increment(x=w379) -> (x+1=w383:u32)
                  n181 = Equal?(x=w379, y=w381) -> (x = y?=w380:bool)
                  n182 = xnode ("Memory Read")("Address"=w379) -> ("Data"=w378:i16)  [unwired: 1 in, 1 out]
                  n183 = Select(t=w377, s=w380, f=w383) -> (s? t:f=w382:u32)
                  n184 = call "Loop Timer16"("Count(Ticks)"=w376) -> ()  [unwired: 1 out]
                  n185 = local read "Start Waveforms"() -> (w375:bool)
                  n186 = xnode "FPGA I/O Node"("Connector0/AO6"=w378) -> ()  [unwired: 1 in, 1 out]
                }
                n187 = timed-loop {
                  timing: w337 -> [_]
                  timing-out: [_] -> w336
                  tunnel: w333 -> [w359]
                  tunnel: [w359] -> w335
                  tunnel: w340 -> [w360]
                  i -> [w362]
                  stop <- w361 stop-if-true
                  n188 = Equal?(x=w360, y=w362) -> (x = y?=w361:bool)
                }
                n189 = while {
                  shift-right: [w350] -> _
                  shift-left: w334 -> [w355]
                  tunnel: w341 -> [w357]
                  tunnel: w335 -> [w353]
                  tunnel: w334 -> [w352]
                  stop <- w351 continue-if-true
                  n190 = Increment(x=w355) -> (x+1=w358:u32)
                  n191 = Equal?(x=w355, y=w357) -> (x = y?=w356:bool)
                  n192 = xnode ("Memory Read")("Address"=w355) -> ("Data"=w354:i16)  [unwired: 1 in, 1 out]
                  n193 = Select(t=w352, s=w356, f=w358) -> (s? t:f=w350:u32)
                  n194 = Less?(x=w350, y=u32 4) -> (x < y?=w348:bool)
                  n195 = local write "Frame Trigger"(w348) -> ()
                  n196 = call "Loop Timer18"("Count(Ticks)"=w353) -> ()  [unwired: 1 out]
                  n197 = xnode "FPGA I/O Node"("Connector0/AO3"=w354) -> ()  [unwired: 1 in, 1 out]
                  n198 = local read "Start Waveforms"() -> (w351:bool)
                }
                n199 = node-c288(w338) -> ()
                n200 = node-c288(w336) -> ()
              }
              frame 6 {
                n201 = node-c288() -> (w405:T4)  [unwired: 1 in]
                n202 = while {
                  tunnel: w402 -> [_]
                  tunnel: w401 -> [w421]
                  tunnel: w398 -> [w422]
                  tunnel: w400 -> [w425]
                  tunnel: w395 -> [w427]
                  stop <- w428 continue-if-true
                  n203 = Quotient & Remainder(x="Current Frame", y=w425) -> (x-y*floor(x/y)=w420:u8)  [unwired: 1 out]
                  n204 = To Word Integer(number=w420) -> (16bit integer=w419:i16)
                  n205 = call "Loop Timer21"("Count(Ticks)"=w427) -> ()  [unwired: 1 out]
                  n206 = Multiply(x=w421, y=w419) -> (x*y=w424:i16)
                  n207 = Add(x=w424, y=w422) -> (x+y=w423:i16)
                  n208 = local read "Start Waveforms"() -> (w428:bool)
                  n209 = xnode "FPGA I/O Node"("Connector0/AO3"=w423) -> ()  [unwired: 1 in, 1 out]
                }
                n210 = while {
                  tunnel: w397 -> [w418]
                  tunnel: w403 -> [w417]
                  tunnel: w395 -> [w416]
                  shift-right: [w414] -> _
                  shift-left: w397 -> [w415]
                  stop <- w408 continue-if-true
                  n211 = Increment(x=w415) -> (x+1=w413:u32)
                  n212 = Equal?(x=w415, y=w417) -> (x = y?=w411:bool)
                  n213 = xnode ("Memory Read")("Address"=w415) -> ("Data"=w412:i16)  [unwired: 1 in, 1 out]
                  n214 = Select(t=w418, s=w411, f=w413) -> (s? t:f=w414:u32)
                  n215 = call "Loop Timer19"("Count(Ticks)"=w416) -> ()  [unwired: 1 out]
                  n216 = Less?(x=w414, y=u32 4) -> (x < y?=w409:bool)
                  n217 = local write "Frame Trigger"(w409) -> ()
                  n218 = xnode "FPGA I/O Node"("Connector0/AO5"=w412) -> ()  [unwired: 1 in, 1 out]
                  n219 = local read "Start Waveforms"() -> (w408:bool)
                }
                n220 = timed-loop {
                  timing: w405 -> [_]
                  timing-out: [_] -> w404
                  tunnel: w395 -> [w440]
                  tunnel: [w440] -> w396
                  tunnel: w406 -> [w441]
                  i -> [w443]
                  stop <- w442 stop-if-true
                  n221 = Equal?(x=w441, y=w443) -> (x = y?=w442:bool)
                }
                n222 = while {
                  shift-right: [w431] -> _
                  shift-left: w397 -> [w437]
                  tunnel: w407 -> [w438]
                  tunnel: w396 -> [w435]
                  tunnel: w397 -> [w434]
                  tunnel: w399 -> [w430]
                  stop <- w433 continue-if-true
                  n223 = Increment(x=w437) -> (x+1=w439:u32)
                  n224 = Equal?(x=w437, y=w438) -> (x = y?=w432:bool)
                  n225 = xnode ("Memory Read")("Address"=w437) -> ("Data"=w436:i16)  [unwired: 1 in, 1 out]
                  n226 = Select(t=w434, s=w432, f=w439) -> (s? t:f=w431:u32)
                  n227 = Greater?(x=w430, y=w431) -> (0:→"End Linear Ramp":bool)
                  n228 = call "Loop Timer20"("Count(Ticks)"=w435) -> ()  [unwired: 1 out]
                  n229 = local read "Start Waveforms"() -> (w433:bool)
                  n230 = xnode "FPGA I/O Node"("Connector0/AO6"=w436) -> ()  [unwired: 1 in, 1 out]
                }
                n231 = node-c288(w404) -> ()
              }
              frame 7 {
                w457 = u8 0
                n232 = node-c288() -> (w462:T4)  [unwired: 1 in]
                n233 = while {
                  shift-right: [w510] -> _
                  shift-left: w463 -> [w516]
                  tunnel: w450 -> [w517]
                  tunnel: w451 -> [w514]
                  tunnel: w463 -> [w513]
                  stop <- w512 continue-if-true
                  n234 = Increment(x=w516) -> (x+1=w518:u32)
                  n235 = Equal?(x=w516, y=w517) -> (x = y?=w511:bool)
                  n236 = xnode ("Memory Read")("Address"=w516) -> ("Data"=w515:i16)  [unwired: 1 in, 1 out]
                  n237 = Select(t=w513, s=w511, f=w518) -> (s? t:f=w510:u32)
                  n238 = call "Loop Timer4"("Count(Ticks)"=w514) -> ()  [unwired: 1 out]
                  n239 = Less?(x=w510, y=u32 20) -> (x < y?=w508:bool)
                  n240 = xnode "FPGA I/O Node"("TRIG0"=w508) -> ()  [unwired: 1 in, 1 out]
                  n241 = local read "Start Waveforms"() -> (w512:bool)
                  n242 = xnode "FPGA I/O Node"("Connector0/AO1"=w515) -> ()  [unwired: 1 in, 1 out]
                }
                n243 = while {
                  shift-right: [w464] -> _
                  shift-left: FALSE -> [w487]
                  shift-right: [w481] -> _
                  shift-left: w457 -> [w483]
                  tunnel: w459 -> [w482]
                  shift-right: [w465] -> _
                  shift-left: w455 -> [w478]
                  tunnel: w458 -> [w477]
                  shift-right: [w471] -> _
                  shift-left: w457 -> [w474]
                  tunnel: w456 -> [w470]
                  tunnel: w455 -> [w467]
                  tunnel: w452 -> [w466]
                  stop <- w488 continue-if-true
                  n244 = local read "End Linear Ramp"() -> (w464:bool)
                  n245 = Increment(x=w483) -> (x+1=w486:u8)
                  n246 = Greater?(x=w464, y=w487) -> (0:w485:bool)
                  n247 = Select(t=w486, s=w485, f=w483) -> (s? t:f=w480:u8)
                  n248 = Add(x=w477, y=w478) -> (x+y=w479:i16)
                  n249 = Increment(x=w474) -> (x+1=w475:u8)
                  n250 = Equal?(x=w480, y=w482) -> (x = y?=w476:bool)
                  n251 = Select(t=u8 0, s=w476, f=w480) -> (s? t:f=w481:u8)
                  n252 = Select(t=w475, s=w476, f=w474) -> (s? t:f=w472:u8)
                  n253 = Select(t=w479, s=w476, f=w478) -> (s? t:f=w473:i16)
                  n254 = call "Loop Timer17"("Count(Ticks)"=w466) -> ()  [unwired: 1 out]
                  n255 = Equal?(x=w472, y=w470) -> (x = y?=w469:bool)
                  n256 = local read "Start Waveforms"() -> (w488:bool)
                  n257 = Select(t=w467, s=w469, f=w473) -> (s? t:f=w465:i16)
                  n258 = xnode "FPGA I/O Node"("Connector0/AO3"=w465) -> ()  [unwired: 1 in, 1 out]
                  n259 = Select(t=u8 0, s=w469, f=w472) -> (s? t:f=w471:u8)
                }
                n260 = timed-loop {
                  timing: w462 -> [_]
                  timing-out: [_] -> w461
                  tunnel: w452 -> [w500]
                  tunnel: [w500] -> w453
                  tunnel: w449 -> [w501]
                  i -> [w503]
                  stop <- w502 stop-if-true
                  n261 = Equal?(x=w501, y=w503) -> (x = y?=w502:bool)
                }
                n262 = while {
                  shift-right: [w491] -> _
                  shift-left: w463 -> [w497]
                  tunnel: w448 -> [w498]
                  tunnel: w453 -> [w495]
                  tunnel: w463 -> [w494]
                  tunnel: w454 -> [w490]
                  stop <- w493 continue-if-true
                  n263 = Increment(x=w497) -> (x+1=w499:u32)
                  n264 = Equal?(x=w497, y=w498) -> (x = y?=w492:bool)
                  n265 = xnode ("Memory Read")("Address"=w497) -> ("Data"=w496:i16)  [unwired: 1 in, 1 out]
                  n266 = Select(t=w494, s=w492, f=w499) -> (s? t:f=w491:u32)
                  n267 = Greater?(x=w490, y=w491) -> (0:w489:bool)
                  n268 = local write "End Linear Ramp"(w489) -> ()
                  n269 = call "Loop Timer15"("Count(Ticks)"=w495) -> ()  [unwired: 1 out]
                  n270 = local read "Start Waveforms"() -> (w493:bool)
                  n271 = xnode "FPGA I/O Node"("Connector0/AO2"=w496) -> ()  [unwired: 1 in, 1 out]
                }
                n272 = node-c288(w461) -> ()
              }
            }
            n273 = case shown="3" w79 {
              frame 0, Default {
              }
              frame 3 {
                n274 = while {
                  stop <- w140 continue-if-true
                  n275 = local read "Start Waveforms"() -> (w140:bool)
                  n276 = xnode "FPGA I/O Node"("Connector0/AO1"="X Piezo Axis", "Connector0/AO2"="Y Piezo Axis", "Connector0/AO3"="Z Piezo Axis") -> ()  [unwired: 3 in, 3 out]
                }
              }
            }
            n277 = Index Array(array="Accums Per Line", index #1=0 ("index"), index #2=1 ("index"), index #3=2 ("index"), index #4=3 ("index")) -> (element #1=w85:u32, element #2=w84:u32, element #3=w83:u32, element #4=w82:u32)
            n278 = Compound Arithmetic op=ADD(w85, w84, w83, w82) -> (w92:u32)
            n279 = Multiply(x="Number of Lines", y=w92) -> (x*y=w93:u32)
            n280 = node-c288() -> (w95:T4)  [unwired: 1 in]
            n281 = timed-loop {
              timing: w95 -> [_]
              timing-out: [_] -> w94
              shift-right: [w129] -> _
              shift-left: w81 -> [w109]
              shift-right: [w127] -> _
              shift-left: _ -> [w110]
              shift-right: [w128] -> _
              shift-left: _ -> [w126]
              shift-right: [w113] -> _
              shift-left: u32 0 -> [w118]
              shift-right: [w122] -> _
              shift-left: w81 -> [w120]
              tunnel: w93 -> [w117]
              tunnel: w79 -> [w111]
              stop <- "Stop Sync Signal" continue-if-true
              n282 = Increment(x=w118) -> (x+1=w121:u32)
              n283 = Equal?(x=w118, y=w117) -> (x = y?=w115:bool)
              n284 = And(x=w110, y=w120) -> (x .and. y?=w125:bool)
              n285 = And(x=w120, y=w110) -> (x .and. y?=w119:bool)
              n286 = local read "Frame Trigger"() -> (w124:bool)
              n287 = Select(t=w121, s=w119, f=w118) -> (s? t:f=w116:u32)
              n288 = case shown="True" w126 {
                tunnel: w125 -> [_ w132]
                frame False {
                }
                frame True {
                  n289 = xnode "FPGA I/O Node"("TRIG1"=w132) -> ()  [unwired: 1 in, 1 out]
                  "Laser Blank Trigger" <- w132
                }
              }
              n290 = xnode ("Register Write")("Data"=w109) -> ()  [unwired: 1 in, 1 out]
              n291 = case shown="0, Default" w111 {
                tunnel: [w130 w131] -> w129
                frame 0, Default {
                  n292 = xnode "FPGA I/O Node"() -> ("Connector1/DIO0"=w130:bool)  [unwired: 1 in, 1 out]
                }
                frame 5 {
                  n293 = xnode ("Register Read")() -> ("Data"=w131:bool)  [unwired: 1 in, 1 out]
                }
              }
              n294 = Exclusive Or(1:w115, 2:w124) -> (0:w123:bool)
              n295 = Select(t=w124, s=w123, f=w120) -> (s? t:f=w122:bool)
              n296 = Select(t=u32 0, s=w115, f=w116) -> (s? t:f=w113:u32)
              n297 = Not Equal?(x=w129, y=w109) -> (x != y?=w128:bool)
              n298 = Greater?(x=w129, y=w109) -> (0:w127:bool)
            }
            n299 = node-c288(w94) -> ()
          }
        }
      }
    }
  }
  n300 = local read "Accums Per Line"() -> (w1:u32[])
  n301 = while {
    shift-right: [w562] -> _
    shift-left: u8 0 -> [w539]
    shift-right: [w563] -> _
    shift-left: w2 -> [w567]
    shift-right: [w561] -> _
    shift-left: u8 0 -> [w564]
    tunnel: "Sequences" -> [w560]
    shift-right: [w554] -> _
    shift-left: u32 0 -> [w555]
    tunnel: w1 -> [w541]
    shift-right: [w521] -> _
    shift-left: w2 -> [w536]
    stop <- FALSE stop-if-true
    n302 = local read "Laser Blank Trigger"() -> (w521:bool)
    n303 = To Long Integer(number=w539) -> (32bit integer=w538:i32)
    n304 = Add(x="Laser Delay (Ticks)", y="Laser On Time (Ticks)") -> (x+y=w525:u8)
    n305 = Index Array(array=w541, index=w538) -> (element=w540:u32)
    n306 = Increment(x=w555) -> (x+1=w556:u32)
    n307 = Equal?(x=w555, y=w540) -> (x = y?=w552:bool)
    n308 = Equal?(x=w564, y=w525) -> (x = y?=w553:bool)
    n309 = Greater?(x=w521, y=w536) -> (0:w535:bool)
    n310 = Select(t=w556, s=w553, f=w555) -> (s? t:f=w557:u32)
    n311 = Increment(x=w539) -> (x+1=w572:u8)
    n312 = Equal?(x=w539, y=w560) -> (x = y?=w569:bool)
    n313 = Exclusive Or(1:w553, 2:w535) -> (0:w568:bool)
    n314 = Select(t=u32 0, s=w552, f=w557) -> (s? t:f=w554:u32)
    n315 = Select(t=w572, s=w552, f=w539) -> (s? t:f=w571:u8)
    n316 = Increment(x=w564) -> (x+1=w566:u8)
    n317 = Select(t=w535, s=w568, f=w567) -> (s? t:f=w563:bool)
    n318 = Split Number(x="Laser States") -> (hi(x)=w549:u16, lo(x)=w550:u16)
    n319 = Select(t=u8 0, s=w569, f=w571) -> (s? t:f=w562:u8)
    n320 = Select(t=w566, s=w563, f=u8 0) -> (s? t:f=w561:u8)
    n321 = Split Number(x=w549) -> (hi(x)=w548:u8, lo(x)=w547:u8)
    n322 = Split Number(x=w550) -> (hi(x)=w546:u8, lo(x)=w545:u8)
    n323 = Greater?(x=w561, y="Laser Delay (Ticks)") -> (0:w537:bool)
    n324 = call "Loop Timer22"("Count(Ticks)"=u16 80) -> ()  [unwired: 1 out]
    n325 = case shown="0, Default" w562 {
      tunnel: w548 -> [w573 _ _ _]
      tunnel: w547 -> [_ w574 _ _]
      tunnel: w546 -> [_ _ w575 _]
      tunnel: w545 -> [_ _ _ w576]
      tunnel: [w573 w574 w575 w576] -> w544
      frame 0, Default {
      }
      frame 1 {
      }
      frame 2 {
      }
      frame 3 {
      }
    }
    n326 = Or(x="Blanking Off/Manual", y=w537) -> (x .or. y?=w520:bool)
    n327 = Select(t=w544, s=w520, f=u8 0) -> (s? t:f=w532:u8)
    n328 = Number To Boolean Array(number=w532) -> (Boolean array=w534:bool[])
    n329 = xnode "FPGA I/O Node"("Connector1/DIO4"="Blanking Off/Manual") -> ()  [unwired: 1 in, 1 out]
    n330 = Index Array(array=w534, index #1=0 ("index"), index #2=1 ("index"), index #3=2 ("index"), index #4=3 ("index")) -> (element #1=w528:bool, element #2=w527:bool, element #3=w523:bool, element #4=w522:bool)
    n331 = xnode "FPGA I/O Node"("Connector0/DIO0"=w528, "Connector1/DIO8"=w527, "Connector1/DIO9"=w523, "Connector1/DIO10"=w522) -> ()  [unwired: 4 in, 4 out]
  }
  n332 = while {
    stop <- "stop" stop-if-true
    n333 = call "Loop Timer23"("Count(uSec)"=u32 100) -> ()  [unwired: 1 out]
    n334 = xnode "FPGA I/O Node"("Connector1/DIO26"="Lower Shutter Command", "Connector1/DIO28"="Upper Shutter Command") -> ("Connector1/DIO25"=→"Lower Shutter Status":bool, "Connector1/DIO27"=→"Upper Shutter Status":bool)  [unwired: 4 in, 4 out]
  }
